vi "Lighthouse Monitoring & Control System with addtional features DONE(GUI LEFT).vi"() -> ()   [LabVIEW 2012]
uses:
  <vilib>/DAQmx/read.llb/DAQmx Read (Counter DBL 1Chan 1Samp).vi
  <vilib>/DAQmx/write.llb/DAQmx Write (Analog DBL 1Chan 1Samp).vi
  <vilib>/DAQmx/write.llb/DAQmx Write (Digital U8 1Chan 1Samp).vi
  <vilib>/DAQmx/write.llb/DAQmx Write (Digital 1D Bool NChan 1Samp 1Line).vi
  <vilib>/DAQmx/read.llb/DAQmx Read (Analog DBL 1Chan 1Samp).vi
  <vilib>/DAQmx/create/channels.llb/DAQmx Create Channel (CI-Count Edges).vi
  <vilib>/DAQmx/create/channels.llb/DAQmx Create Channel (DO-Digital Output).vi
  <vilib>/DAQmx/create/channels.llb/DAQmx Create Channel (AI-Voltage-Basic).vi
  <vilib>/DAQmx/create/channels.llb/DAQmx Create Channel (AO-Voltage-Basic).vi
  <vilib>/DAQmx/miscellaneous.llb/DAQmx Fill In Error Info.vi
panel:
  out "Voltage":dbl
  out "Slot Count":dbl
  out "Data to Write":u32=255 format="%x"
  out "Motor":bool[](array[boolean])
  out "LED 3":bool
  out "LED 2":bool
  out "LED 1":bool
  in  "?":bool
  in  "Switch":bool
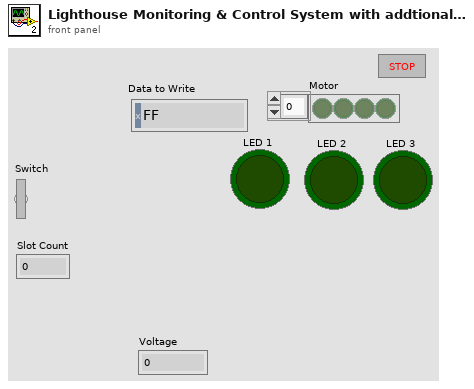
[diagram p1: front panel]
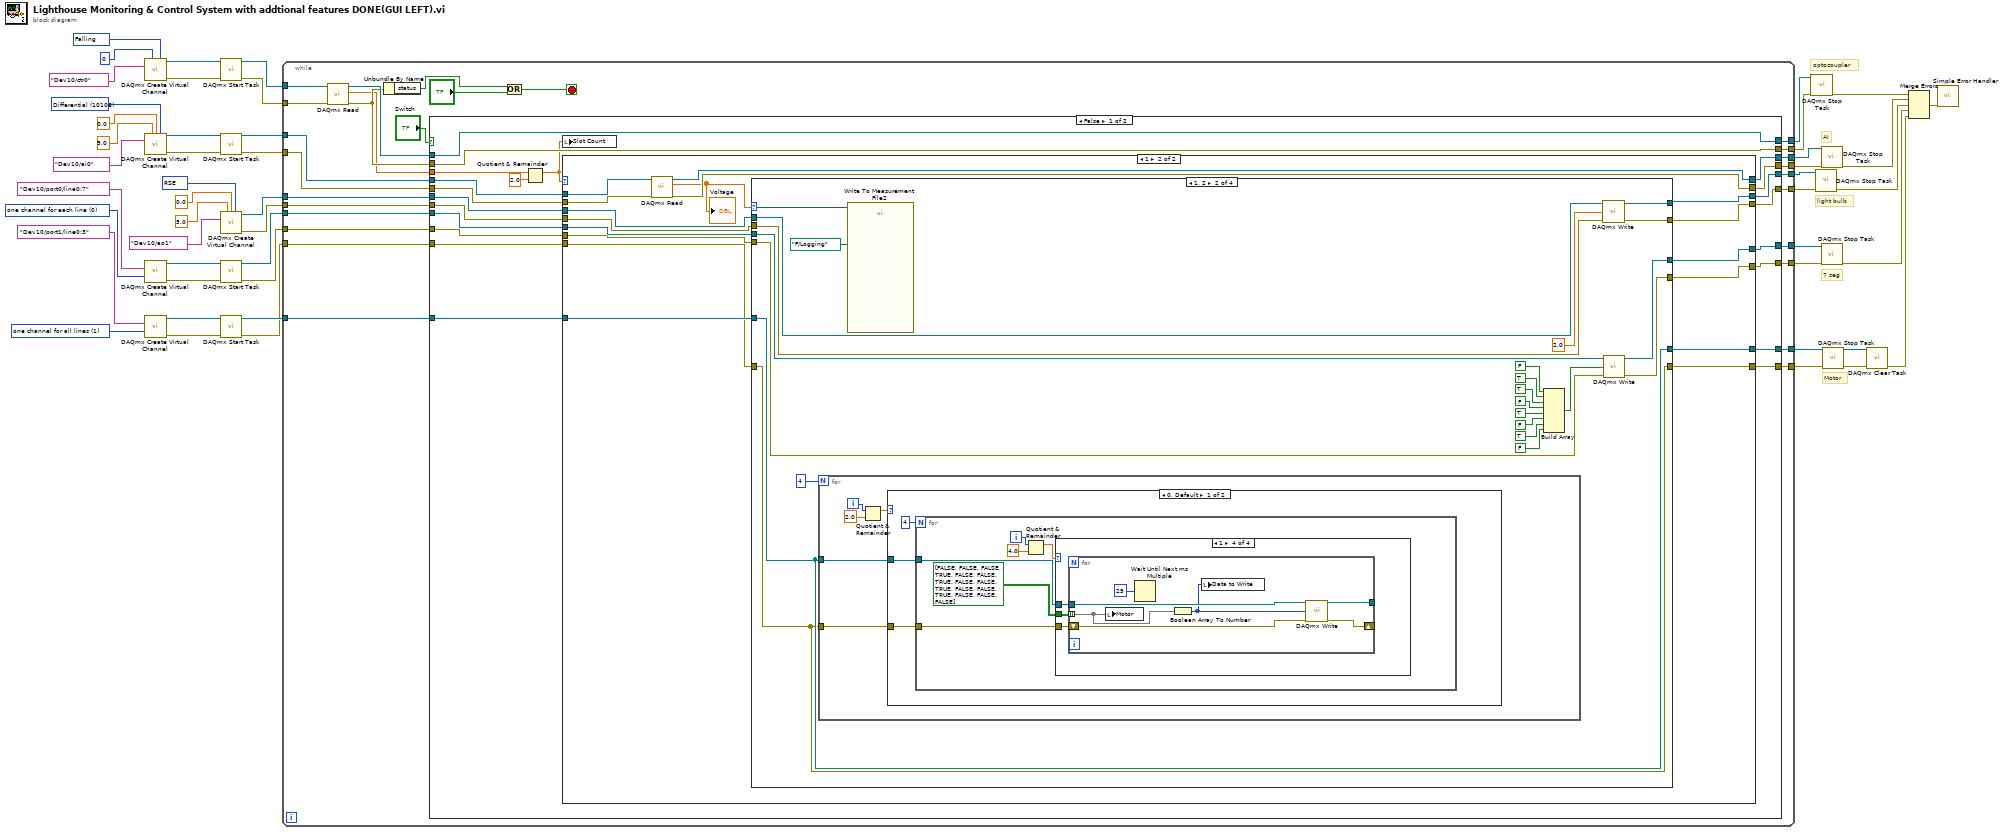
[diagram p0: block diagram]
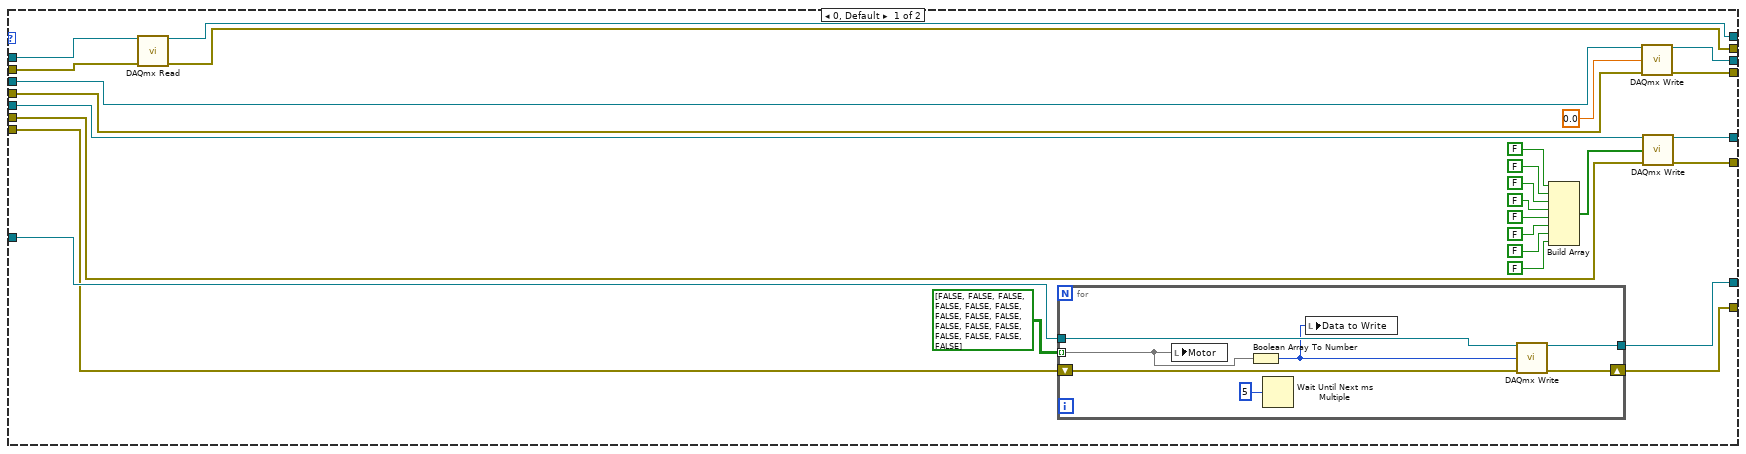
[diagram p2: hidden frame]
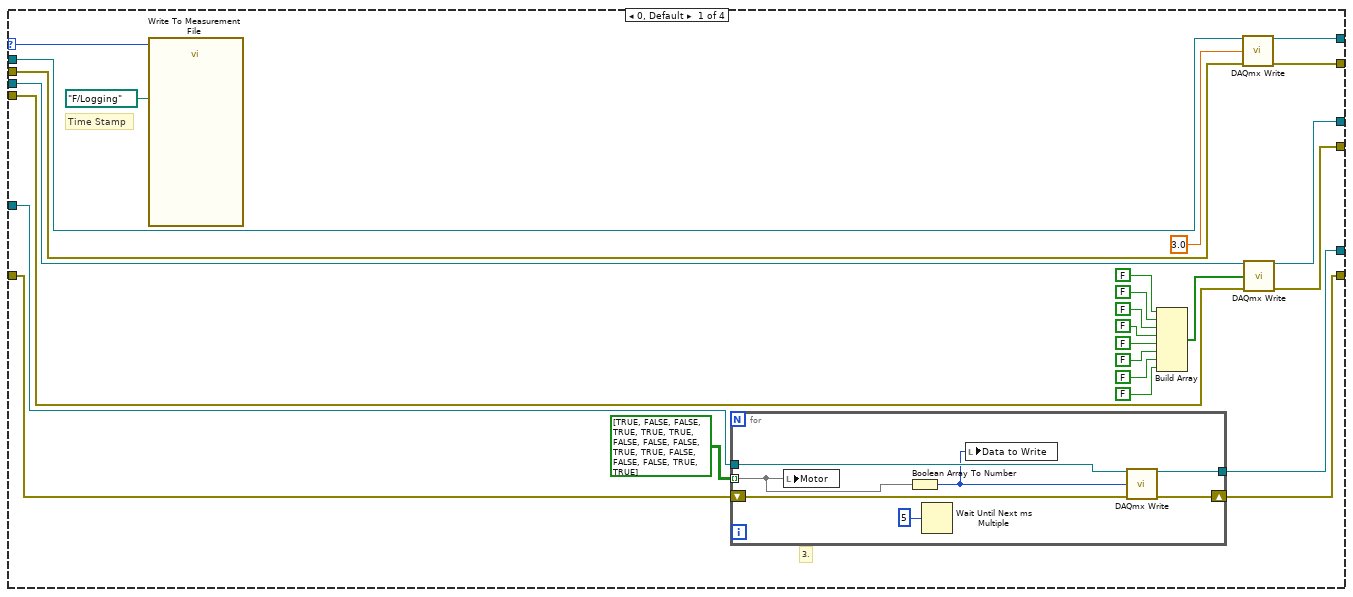
[diagram p3: hidden frame]
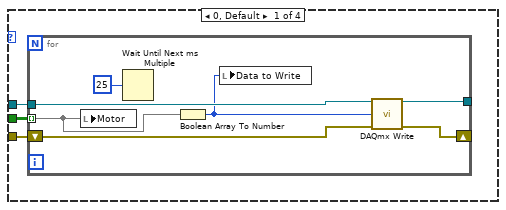
[diagram p4: hidden frame]
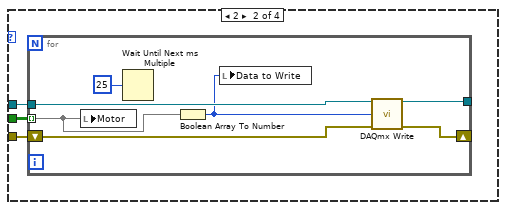
[diagram p5: hidden frame]
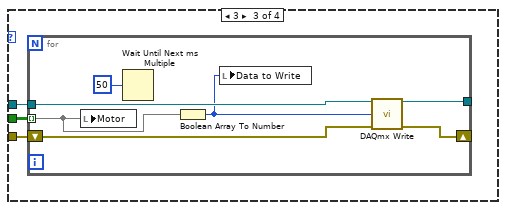
[diagram p6: hidden frame]
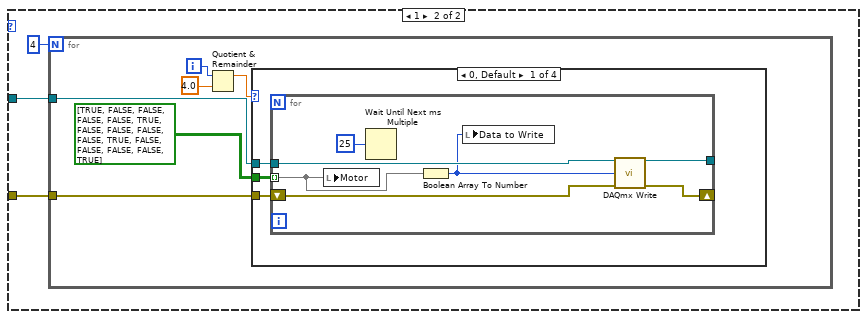
[diagram p7: hidden frame]
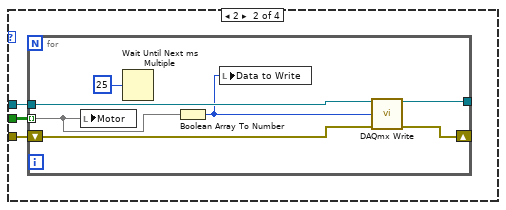
[diagram p8: hidden frame]
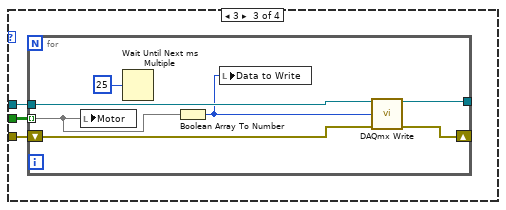
[diagram p9: hidden frame]
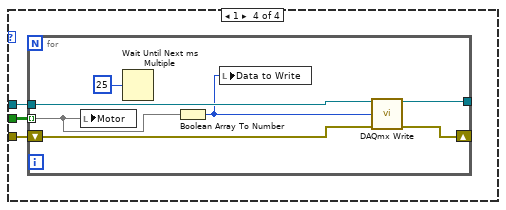
[diagram p10: hidden frame]
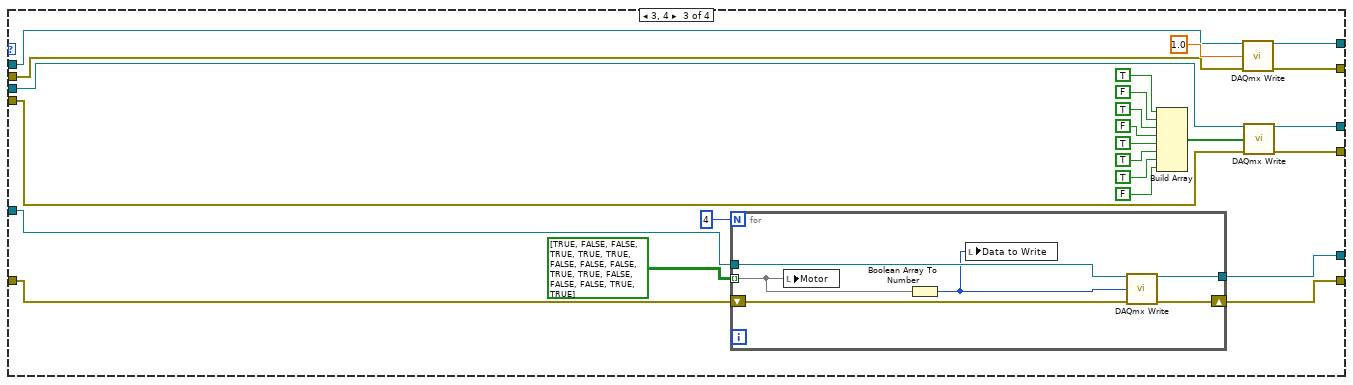
[diagram p11: hidden frame]
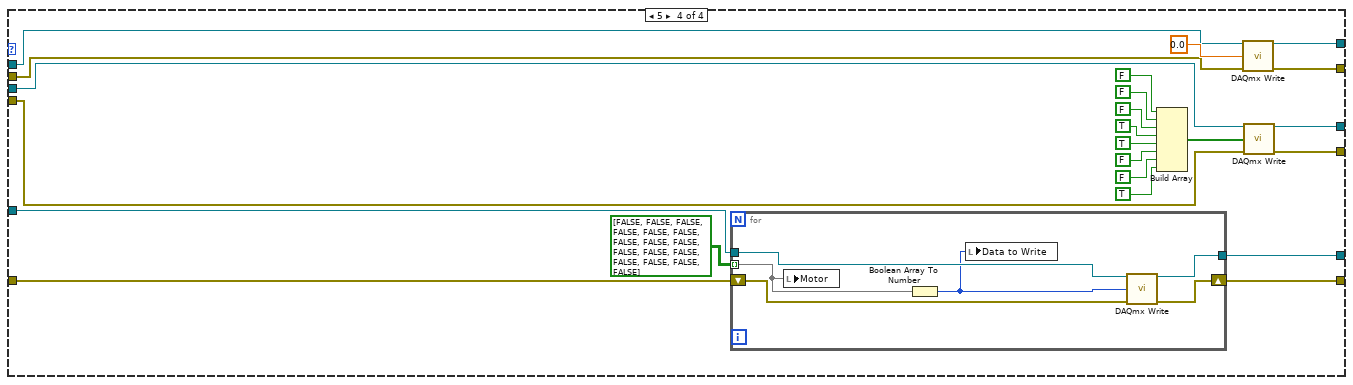
[diagram p12: hidden frame]
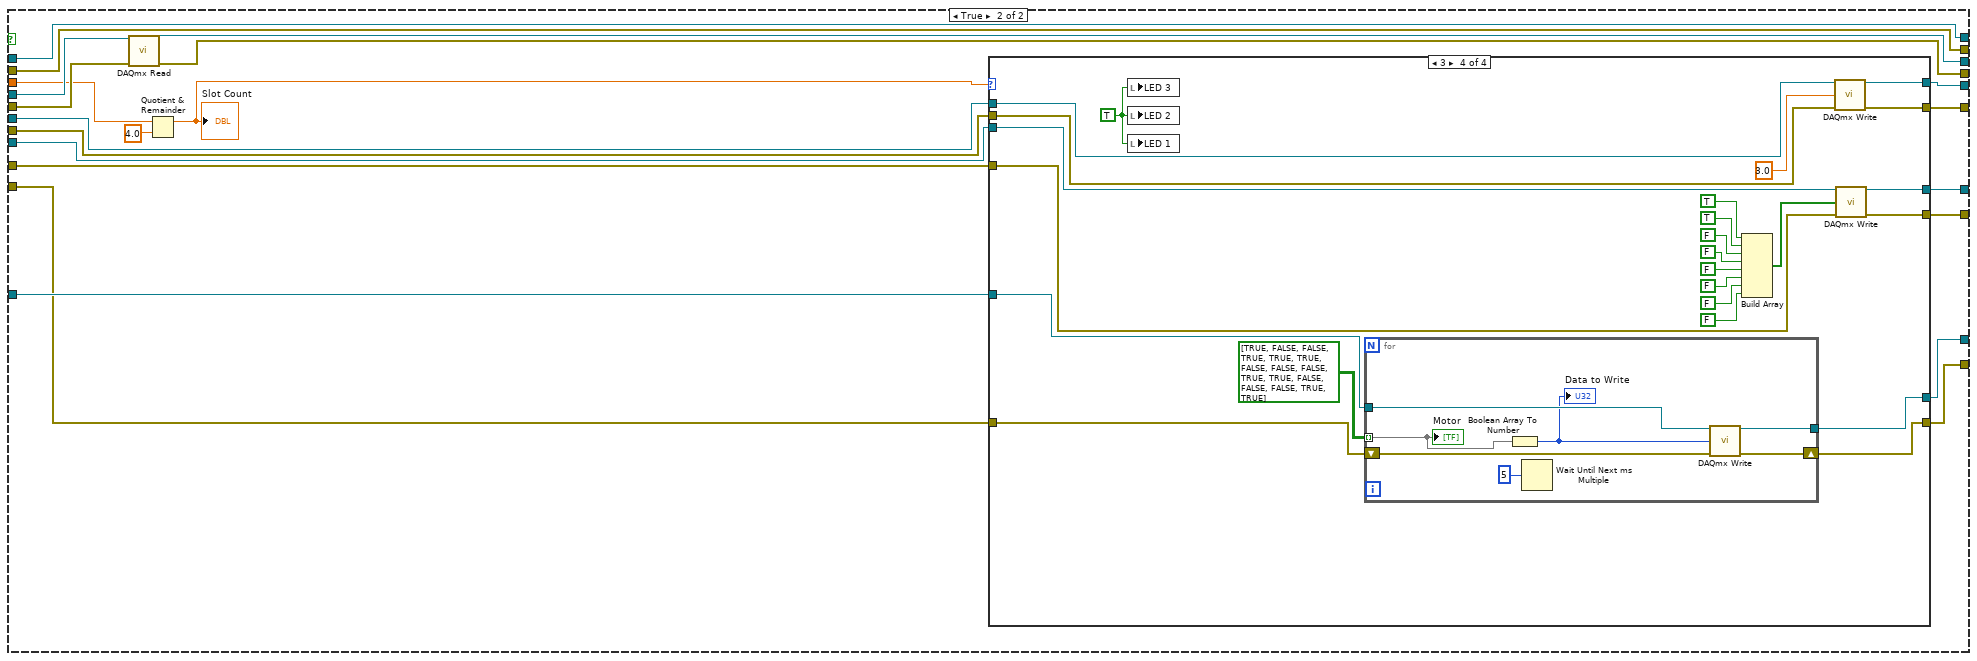
[diagram p13: hidden frame]
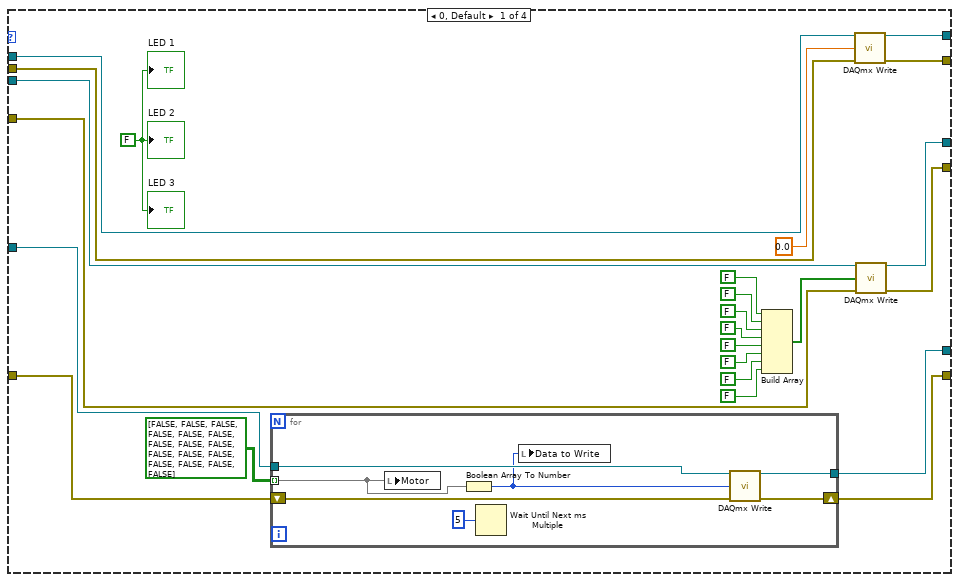
[diagram p14: hidden frame]
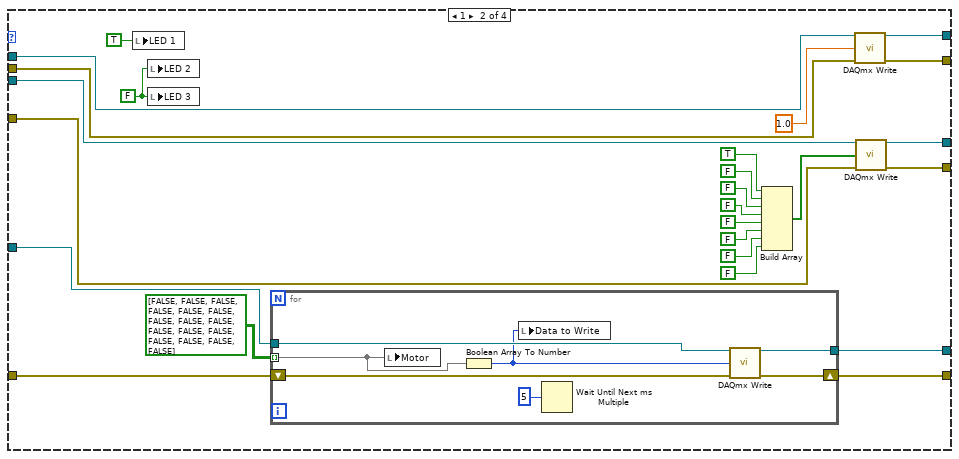
[diagram p15: hidden frame]
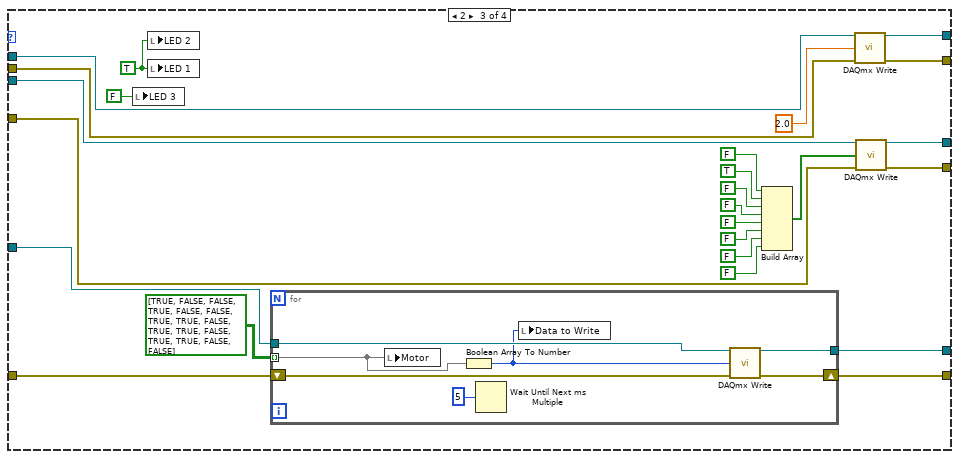
[diagram p16: hidden frame]
diagram:
  w24 = 10083 items=["Default"=-1, "RSE"=10083, "Differential"=10106, "Pseudodifferential"=12529] ("output terminal configuration")
  w32 = 10106 items=["default"=-1, "RSE"=10083, "NRSE"=10078, "Differential"=10106, "Pseudodifferential"=12529] ("input terminal configuration")
  w42 = 1 items=["one channel for each line", "one channel for all lines"] ("line grouping")
  w37 = 0 items=["one channel for each line", "one channel for all lines"] ("line grouping")
  w51 = 10171 items=["Rising"=10280, "Falling"=10171] ("edge")
  # "Motor"
  # "7 seg"
  # "AI"
  # "light bulb"
  # "optocoupler"
  n1 = call-poly <vilib>:"DAQmx Create Virtual Channel.vi"("initial count"=u32 0, "edge"=w51, "counter"=tag "Dev10/ctr0") -> ("task out"=w50:refnum<k21>, "error out"=w49:errorcluster)  [unwired: 11 in]
  n2 = call-poly <vilib>:"DAQmx Create Virtual Channel.vi"("maximum value"=5.0, "minimum value"=0.0, "input terminal configuration"=w32, "physical channels"=tag "Dev10/ai0") -> ("task out"=w30:refnum<k21>, "error out"=w31:errorcluster)  [unwired: 10 in]
  n3 = call-poly <vilib>:"DAQmx Create Virtual Channel.vi"("lines"=tag "Dev10/port0/line0:7", "line grouping"=w37) -> ("task out"=w44:refnum<k21>, "error out"=w43:errorcluster)  [unwired: 12 in]
  n4 = call-poly <vilib>:"DAQmx Create Virtual Channel.vi"("lines"=tag "Dev10/port1/line0:3", "line grouping"=w42) -> ("task out"=w41:refnum<k21>, "error out"=w40:errorcluster)  [unwired: 12 in]
  n5 = call <vilib>:"DAQmx Start Task.vi"("task/channels in"=w50, "error in"=w49) -> ("task out"=w46:refnum<k21>, "error out"=w45:errorcluster)  [unwired: 12 in]
  n6 = call <vilib>:"DAQmx Start Task.vi"("task/channels in"=w30, "error in"=w31) -> ("task out"=w26:refnum<k21>, "error out"=w25:errorcluster)  [unwired: 12 in]
  n7 = call-poly <vilib>:"DAQmx Create Virtual Channel.vi"("maximum value"=5.0, "minimum value"=0.0, "output terminal configuration"=w24, "physical channels"=tag "Dev10/ao1") -> ("task out"=w20:refnum<k21>, "error out"=w19:errorcluster)  [unwired: 10 in]
  n8 = call <vilib>:"DAQmx Start Task.vi"("task/channels in"=w44, "error in"=w43) -> ("task out"=w36:refnum<k21>, "error out"=w35:errorcluster)  [unwired: 12 in]
  n9 = call <vilib>:"DAQmx Start Task.vi"("task/channels in"=w41, "error in"=w40) -> ("task out"=w34:refnum<k21>, "error out"=w33:errorcluster)  [unwired: 12 in]
  n10 = while {
    tunnel: w46 -> [w77]
    tunnel: w45 -> [w76]
    tunnel: w36 -> [w75]
    tunnel: w35 -> [w74]
    tunnel: w34 -> [w73]
    tunnel: w33 -> [w72]
    tunnel: w26 -> [w70]
    tunnel: w25 -> [w69]
    tunnel: w20 -> [w68]
    tunnel: w19 -> [w67]
    tunnel: [w61] -> w10
    tunnel: [w60] -> w9
    tunnel: [w59] -> w8
    tunnel: [w58] -> w7
    tunnel: [w57] -> w6
    tunnel: [w56] -> w5
    tunnel: [w55] -> w4
    tunnel: [w54] -> w3
    tunnel: [w53] -> w2
    tunnel: [w52] -> w1
    stop <- w62 stop-if-true
    n11 = call-poly <vilib>:"DAQmx Read.vi"("task/channels in"=w77, "error in"=w76) -> ("task out"=w65:refnum<k21>, "data"=w63:dbl, "error out"=w64:errorcluster)  [unwired: 11 in]
    n12 = Unbundle By Name(w64) -> ("status"=w71:bool)
    n13 = case shown="False" "Switch" {
      tunnel: w75 -> [w87 w388]
      tunnel: w74 -> [w86 w387]
      tunnel: w73 -> [w85 w386]
      tunnel: w72 -> [w84 w385]
      tunnel: [w83 w384] -> w55
      tunnel: [w82 w383] -> w54
      tunnel: w70 -> [w97 w380]
      tunnel: w69 -> [w96 w379]
      tunnel: w68 -> [w81 w382]
      tunnel: w67 -> [w80 w381]
      tunnel: [w95 w378] -> w53
      tunnel: [w94 w377] -> w52
      tunnel: [w93 w376] -> w59
      tunnel: [w92 w375] -> w58
      tunnel: [w89 w374] -> w56
      tunnel: [w88 w373] -> w57
      tunnel: w65 -> [w91 w369]
      tunnel: w64 -> [w90 w368]
      tunnel: w63 -> [w98 w371]
      tunnel: [w91 w369] -> w61
      tunnel: [w90 w368] -> w60
      frame False {
        n14 = Quotient & Remainder(x=w98, y=2.0) -> (x-y*floor(x/y)=w79:dbl)  [unwired: 1 out]
        n15 = local write "Slot Count"(w79) -> ()
        n16 = case shown="1" w79 {
          tunnel: w97 -> [w125 w150]
          tunnel: w96 -> [w124 w149]
          tunnel: [w121 w148] -> w93
          tunnel: [w122 w147] -> w92
          tunnel: [w123 w146] -> w94
          tunnel: [w118 w145] -> w89
          tunnel: [w119 w144] -> w88
          tunnel: [w120 w143] -> w95
          tunnel: [w106 w141] -> w82
          tunnel: [w107 w142] -> w83
          tunnel: w87 -> [w105 w135]
          tunnel: w86 -> [w104 w134]
          tunnel: w85 -> [w103 w137]
          tunnel: w84 -> [w102 w136]
          tunnel: w81 -> [w101 w139]
          tunnel: w80 -> [w100 w138]
          frame 0, Default {
            n17 = call-poly <vilib>:"DAQmx Read.vi"("task/channels in"=w125, "error in"=w124) -> ("task out"=w120:refnum<k21>, "error out"=w123:errorcluster)  [unwired: 11 in, 1 out]
            n18 = for {
              tunnel: [w132] -> w107
              shift-right: [w130] -> w106
              shift-left: w102 -> [w133]
              tunnel: bool[][] [[FALSE, FALSE, FALSE, FALSE], [FALSE, FALSE, FALSE, FALSE], [FALSE, FALSE, FALSE, FALSE], [FALSE, FALSE, FALSE, FALSE]] -> [w127] mode=indexing
              tunnel: w103 -> [w129]
              n19 = local write "Motor"(w127) -> ()
              n20 = Boolean Array To Number(Boolean array=w127) -> (number=w128:u32)
              n21 = Wait Until Next ms Multiple(millisecond multiple=5) -> ()  [unwired: 1 out]
              n22 = local write "Data to Write"(w128) -> ()
              n23 = call-poly <vilib>:"DAQmx Write.vi"("task/channels in"=w129, "data"=w128, "error in"=w133) -> ("task out"=w132:refnum<k21>, "error out"=w130:errorcluster)  [unwired: 10 in, 1 out]
            }
            n24 = Build Array(FALSE, FALSE, FALSE, FALSE, FALSE, FALSE, FALSE, FALSE) -> (w109:bool[])
            n25 = call-poly <vilib>:"DAQmx Write.vi"("task/channels in"=w101, "data"=0.0, "error in"=w100) -> ("task out"=w121:refnum<k21>, "error out"=w122:errorcluster)  [unwired: 10 in, 1 out]
            n26 = call-poly <vilib>:"DAQmx Write.vi"("task/channels in"=w105, "data"=w109, "error in"=w104) -> ("task out"=w119:refnum<k21>, "error out"=w118:errorcluster)  [unwired: 10 in, 1 out]
          }
          frame 1 {
            n27 = call-poly <vilib>:"DAQmx Read.vi"("task/channels in"=w150, "error in"=w149) -> ("task out"=w143:refnum<k21>, "data"=w140:dbl, "error out"=w146:errorcluster)  [unwired: 11 in]
            "Voltage" <- w140
            n28 = case shown="1, 2" w140 {
              selector: w140 -> [w157 w190 _ _]
              tunnel: [w165 w195 w322 w351] -> w148
              tunnel: [w164 w194 w321 w350] -> w147
              tunnel: [w163 w193 w320 w349] -> w144
              tunnel: [w162 w192 w319 w348] -> w145
              tunnel: [w161 w184 w317 w346] -> w142
              tunnel: [w160 w183 w316 w345] -> w141
              tunnel: w139 -> [w156 w189 w315 w344]
              tunnel: w138 -> [w155 w188 w314 w343]
              tunnel: w137 -> [w154 w184 w311 w340]
              tunnel: w136 -> [w151 w183 w310 w339]
              tunnel: w135 -> [w153 w187 w313 w342]
              tunnel: w134 -> [w152 w186 w312 w341]
              frame 0, Default {
                # "3."
                # "Time Stamp"
                n29 = call "Write To Measurement File"("Signals"=w157, "Filename"=path "F:/Logging") -> ()  [unwired: 15 in, 3 out]
                n30 = for {
                  tunnel: [w181] -> w161
                  shift-right: [w180] -> w160
                  shift-left: w151 -> [w182]
                  tunnel: bool[][] [[TRUE, FALSE, FALSE, TRUE], [TRUE, TRUE, FALSE, FALSE], [FALSE, TRUE, TRUE, FALSE], [FALSE, FALSE, TRUE, TRUE]] -> [w176] mode=indexing
                  tunnel: w154 -> [w178]
                  n31 = local write "Motor"(w176) -> ()
                  n32 = Boolean Array To Number(Boolean array=w176) -> (number=w177:u32)
                  n33 = Wait Until Next ms Multiple(millisecond multiple=u32 5) -> ()  [unwired: 1 out]
                  n34 = local write "Data to Write"(w177) -> ()
                  n35 = call-poly <vilib>:"DAQmx Write.vi"("task/channels in"=w178, "data"=w177, "error in"=w182) -> ("task out"=w181:refnum<k21>, "error out"=w180:errorcluster)  [unwired: 10 in, 1 out]
                }
                n36 = Build Array(FALSE, FALSE, FALSE, FALSE, FALSE, FALSE, FALSE, FALSE) -> (w166:bool[])
                n37 = call-poly <vilib>:"DAQmx Write.vi"("task/channels in"=w156, "data"=3.0, "error in"=w155) -> ("task out"=w165:refnum<k21>, "error out"=w164:errorcluster)  [unwired: 10 in, 1 out]
                n38 = call-poly <vilib>:"DAQmx Write.vi"("task/channels in"=w153, "data"=w166, "error in"=w152) -> ("task out"=w163:refnum<k21>, "error out"=w162:errorcluster)  [unwired: 10 in, 1 out]
              }
              frame 1, 2 {
                n39 = for {
                  N: 4 -> [_]
                  tunnel: w184 -> [w210]
                  tunnel: w183 -> [w209]
                  i -> [w207]
                  n40 = Quotient & Remainder(x=w207, y=2.0) -> (x-y*floor(x/y)=w206:dbl)  [unwired: 1 out]
                  n41 = case shown="0, Default" w206 {
                    tunnel: w210 -> [w213 w262]
                    tunnel: w209 -> [w212 w261]
                    frame 0, Default {
                      n42 = for {
                        N: 4 -> [_]
                        tunnel: w213 -> [w219]
                        tunnel: w212 -> [w218]
                        i -> [w215]
                        n43 = Quotient & Remainder(x=w215, y=4.0) -> (x-y*floor(x/y)=w214:dbl)  [unwired: 1 out]
                        n44 = case shown="1" w214 {
                          tunnel: w219 -> [w222 w232 w241 w252]
                          tunnel: w218 -> [w220 w231 w242 w251]
                          tunnel: bool[][] [[FALSE, FALSE, FALSE, TRUE], [FALSE, FALSE, TRUE, FALSE], [FALSE, TRUE, FALSE, FALSE], [TRUE, FALSE, FALSE, FALSE]] -> [w221 w230 w240 w250]
                          frame 0, Default {
                            n45 = for {
                              tunnel: [w228] -> _
                              shift-right: [w227] -> _
                              shift-left: w220 -> [w229]
                              tunnel: w221 -> [w223] mode=indexing
                              tunnel: w222 -> [w225]
                              n46 = local write "Motor"(w223) -> ()
                              n47 = Wait Until Next ms Multiple(millisecond multiple=u32 25) -> ()  [unwired: 1 out]
                              n48 = Boolean Array To Number(Boolean array=w223) -> (number=w224:u32)
                              n49 = local write "Data to Write"(w224) -> ()
                              n50 = call-poly <vilib>:"DAQmx Write.vi"("task/channels in"=w225, "data"=w224, "error in"=w229) -> ("task out"=w228:refnum<k21>, "error out"=w227:errorcluster)  [unwired: 10 in, 1 out]
                            }
                          }
                          frame 2 {
                            n51 = for {
                              tunnel: [w238] -> _
                              shift-right: [w237] -> _
                              shift-left: w231 -> [w239]
                              tunnel: w230 -> [w233] mode=indexing
                              tunnel: w232 -> [w235]
                              n52 = local write "Motor"(w233) -> ()
                              n53 = Wait Until Next ms Multiple(millisecond multiple=u32 25) -> ()  [unwired: 1 out]
                              n54 = Boolean Array To Number(Boolean array=w233) -> (number=w234:u32)
                              n55 = local write "Data to Write"(w234) -> ()
                              n56 = call-poly <vilib>:"DAQmx Write.vi"("task/channels in"=w235, "data"=w234, "error in"=w239) -> ("task out"=w238:refnum<k21>, "error out"=w237:errorcluster)  [unwired: 10 in, 1 out]
                            }
                          }
                          frame 3 {
                            n57 = for {
                              tunnel: [w248] -> _
                              shift-right: [w247] -> _
                              shift-left: w242 -> [w249]
                              tunnel: w240 -> [w244] mode=indexing
                              tunnel: w241 -> [w245]
                              n58 = local write "Motor"(w244) -> ()
                              n59 = Wait Until Next ms Multiple(millisecond multiple=u32 50) -> ()  [unwired: 1 out]
                              n60 = Boolean Array To Number(Boolean array=w244) -> (number=w243:u32)
                              n61 = local write "Data to Write"(w243) -> ()
                              n62 = call-poly <vilib>:"DAQmx Write.vi"("task/channels in"=w245, "data"=w243, "error in"=w249) -> ("task out"=w248:refnum<k21>, "error out"=w247:errorcluster)  [unwired: 10 in, 1 out]
                            }
                          }
                          frame 1 {
                            n63 = for {
                              tunnel: [w258] -> _
                              shift-right: [w257] -> _
                              shift-left: w251 -> [w259]
                              tunnel: w250 -> [w254] mode=indexing
                              tunnel: w252 -> [w255]
                              n64 = local write "Motor"(w254) -> ()
                              n65 = Wait Until Next ms Multiple(millisecond multiple=u32 25) -> ()  [unwired: 1 out]
                              n66 = Boolean Array To Number(Boolean array=w254) -> (number=w253:u32)
                              n67 = local write "Data to Write"(w253) -> ()
                              n68 = call-poly <vilib>:"DAQmx Write.vi"("task/channels in"=w255, "data"=w253, "error in"=w259) -> ("task out"=w258:refnum<k21>, "error out"=w257:errorcluster)  [unwired: 10 in, 1 out]
                            }
                          }
                        }
                      }
                    }
                    frame 1 {
                      n69 = for {
                        N: 4 -> [_]
                        tunnel: w262 -> [w268]
                        tunnel: w261 -> [w267]
                        i -> [w266]
                        n70 = Quotient & Remainder(x=w266, y=4.0) -> (x-y*floor(x/y)=w264:dbl)  [unwired: 1 out]
                        n71 = case shown="0, Default" w264 {
                          tunnel: w268 -> [w271 w281 w290 w301]
                          tunnel: w267 -> [w270 w280 w291 w300]
                          tunnel: bool[][] [[TRUE, FALSE, FALSE, FALSE], [FALSE, TRUE, FALSE, FALSE], [FALSE, FALSE, TRUE, FALSE], [FALSE, FALSE, FALSE, TRUE]] -> [w269 w279 w289 w299]
                          frame 0, Default {
                            n72 = for {
                              tunnel: [w277] -> _
                              shift-right: [w276] -> _
                              shift-left: w270 -> [w278]
                              tunnel: w269 -> [w273] mode=indexing
                              tunnel: w271 -> [w274]
                              n73 = local write "Motor"(w273) -> ()
                              n74 = Wait Until Next ms Multiple(millisecond multiple=u32 25) -> ()  [unwired: 1 out]
                              n75 = Boolean Array To Number(Boolean array=w273) -> (number=w272:u32)
                              n76 = local write "Data to Write"(w272) -> ()
                              n77 = call-poly <vilib>:"DAQmx Write.vi"("task/channels in"=w274, "data"=w272, "error in"=w278) -> ("task out"=w277:refnum<k21>, "error out"=w276:errorcluster)  [unwired: 10 in, 1 out]
                            }
                          }
                          frame 2 {
                            n78 = for {
                              tunnel: [w287] -> _
                              shift-right: [w286] -> _
                              shift-left: w280 -> [w288]
                              tunnel: w279 -> [w282] mode=indexing
                              tunnel: w281 -> [w284]
                              n79 = local write "Motor"(w282) -> ()
                              n80 = Wait Until Next ms Multiple(millisecond multiple=u32 25) -> ()  [unwired: 1 out]
                              n81 = Boolean Array To Number(Boolean array=w282) -> (number=w283:u32)
                              n82 = local write "Data to Write"(w283) -> ()
                              n83 = call-poly <vilib>:"DAQmx Write.vi"("task/channels in"=w284, "data"=w283, "error in"=w288) -> ("task out"=w287:refnum<k21>, "error out"=w286:errorcluster)  [unwired: 10 in, 1 out]
                            }
                          }
                          frame 3 {
                            n84 = for {
                              tunnel: [w297] -> _
                              shift-right: [w296] -> _
                              shift-left: w291 -> [w298]
                              tunnel: w289 -> [w293] mode=indexing
                              tunnel: w290 -> [w294]
                              n85 = local write "Motor"(w293) -> ()
                              n86 = Wait Until Next ms Multiple(millisecond multiple=u32 25) -> ()  [unwired: 1 out]
                              n87 = Boolean Array To Number(Boolean array=w293) -> (number=w292:u32)
                              n88 = local write "Data to Write"(w292) -> ()
                              n89 = call-poly <vilib>:"DAQmx Write.vi"("task/channels in"=w294, "data"=w292, "error in"=w298) -> ("task out"=w297:refnum<k21>, "error out"=w296:errorcluster)  [unwired: 10 in, 1 out]
                            }
                          }
                          frame 1 {
                            n90 = for {
                              tunnel: [w307] -> _
                              shift-right: [w306] -> _
                              shift-left: w300 -> [w308]
                              tunnel: w299 -> [w303] mode=indexing
                              tunnel: w301 -> [w304]
                              n91 = local write "Motor"(w303) -> ()
                              n92 = Wait Until Next ms Multiple(millisecond multiple=u32 25) -> ()  [unwired: 1 out]
                              n93 = Boolean Array To Number(Boolean array=w303) -> (number=w302:u32)
                              n94 = local write "Data to Write"(w302) -> ()
                              n95 = call-poly <vilib>:"DAQmx Write.vi"("task/channels in"=w304, "data"=w302, "error in"=w308) -> ("task out"=w307:refnum<k21>, "error out"=w306:errorcluster)  [unwired: 10 in, 1 out]
                            }
                          }
                        }
                      }
                    }
                  }
                }
                n96 = call "Write To Measurement File2"("Signals"=w190, "Filename"=path "F:/Logging") -> ()  [unwired: 15 in, 3 out]
                n97 = Build Array(FALSE, TRUE, TRUE, FALSE, TRUE, FALSE, TRUE, FALSE) -> (w196:bool[])
                n98 = call-poly <vilib>:"DAQmx Write.vi"("task/channels in"=w189, "data"=2.0, "error in"=w188) -> ("task out"=w195:refnum<k21>, "error out"=w194:errorcluster)  [unwired: 10 in, 1 out]
                n99 = call-poly <vilib>:"DAQmx Write.vi"("task/channels in"=w187, "data"=w196, "error in"=w186) -> ("task out"=w193:refnum<k21>, "error out"=w192:errorcluster)  [unwired: 10 in, 1 out]
              }
              frame 3, 4 {
                n100 = for {
                  N: 4 -> [_]
                  tunnel: [w337] -> w317
                  shift-right: [w336] -> w316
                  shift-left: w310 -> [w338]
                  tunnel: bool[][] [[TRUE, FALSE, FALSE, TRUE], [TRUE, TRUE, FALSE, FALSE], [FALSE, TRUE, TRUE, FALSE], [FALSE, FALSE, TRUE, TRUE]] -> [w333] mode=indexing
                  tunnel: w311 -> [w335]
                  n101 = local write "Motor"(w333) -> ()
                  n102 = Boolean Array To Number(Boolean array=w333) -> (number=w334:u32)
                  n103 = local write "Data to Write"(w334) -> ()
                  n104 = call-poly <vilib>:"DAQmx Write.vi"("task/channels in"=w335, "data"=w334, "error in"=w338) -> ("task out"=w337:refnum<k21>, "error out"=w336:errorcluster)  [unwired: 10 in, 1 out]
                }
                n105 = Build Array(TRUE, FALSE, TRUE, FALSE, TRUE, TRUE, TRUE, FALSE) -> (w323:bool[])
                n106 = call-poly <vilib>:"DAQmx Write.vi"("task/channels in"=w315, "data"=1.0, "error in"=w314) -> ("task out"=w322:refnum<k21>, "error out"=w321:errorcluster)  [unwired: 10 in, 1 out]
                n107 = call-poly <vilib>:"DAQmx Write.vi"("task/channels in"=w313, "data"=w323, "error in"=w312) -> ("task out"=w320:refnum<k21>, "error out"=w319:errorcluster)  [unwired: 10 in, 1 out]
              }
              frame 5 {
                n108 = for {
                  tunnel: [w366] -> w346
                  shift-right: [w365] -> w345
                  shift-left: w339 -> [w367]
                  tunnel: bool[][] [[FALSE, FALSE, FALSE, FALSE], [FALSE, FALSE, FALSE, FALSE], [FALSE, FALSE, FALSE, FALSE], [FALSE, FALSE, FALSE, FALSE]] -> [w362] mode=indexing
                  tunnel: w340 -> [w364]
                  n109 = local write "Motor"(w362) -> ()
                  n110 = Boolean Array To Number(Boolean array=w362) -> (number=w363:u32)
                  n111 = local write "Data to Write"(w363) -> ()
                  n112 = call-poly <vilib>:"DAQmx Write.vi"("task/channels in"=w364, "data"=w363, "error in"=w367) -> ("task out"=w366:refnum<k21>, "error out"=w365:errorcluster)  [unwired: 10 in, 1 out]
                }
                n113 = Build Array(FALSE, FALSE, FALSE, TRUE, TRUE, FALSE, FALSE, TRUE) -> (w352:bool[])
                n114 = call-poly <vilib>:"DAQmx Write.vi"("task/channels in"=w344, "data"=0.0, "error in"=w343) -> ("task out"=w351:refnum<k21>, "error out"=w350:errorcluster)  [unwired: 10 in, 1 out]
                n115 = call-poly <vilib>:"DAQmx Write.vi"("task/channels in"=w342, "data"=w352, "error in"=w341) -> ("task out"=w349:refnum<k21>, "error out"=w348:errorcluster)  [unwired: 10 in, 1 out]
              }
            }
          }
        }
      }
      frame True {
        n116 = call-poly <vilib>:"DAQmx Read.vi"("task/channels in"=w380, "error in"=w379) -> ("task out"=w378:refnum<k21>, "error out"=w377:errorcluster)  [unwired: 11 in, 1 out]
        n117 = Quotient & Remainder(x=w371, y=4.0) -> (x-y*floor(x/y)=w370:dbl)  [unwired: 1 out]
        "Slot Count" <- w370
        n118 = case shown="3" w370 {
          tunnel: w388 -> [w400 w428 w460 w491]
          tunnel: w387 -> [w399 w427 w461 w492]
          tunnel: w386 -> [w412 w426 w457 w489]
          tunnel: w385 -> [w411 w425 w458 w488]
          tunnel: [w410 w424 w456 w487] -> w384
          tunnel: [w409 w423 w455 w486] -> w383
          tunnel: w382 -> [w397 w439 w473 w504]
          tunnel: w381 -> [w396 w438 w472 w503]
          tunnel: [w395 w441 w475 w506] -> w376
          tunnel: [w394 w440 w474 w505] -> w375
          tunnel: [w391 w421 w453 w485] -> w373
          tunnel: [w390 w420 w452 w484] -> w374
          frame 0, Default {
            w392 = FALSE
            n119 = for {
              tunnel: [w418] -> w410
              shift-right: [w416] -> w409
              shift-left: w411 -> [w419]
              tunnel: w412 -> [w415]
              tunnel: bool[][] [[FALSE, FALSE, FALSE, FALSE], [FALSE, FALSE, FALSE, FALSE], [FALSE, FALSE, FALSE, FALSE], [FALSE, FALSE, FALSE, FALSE]] -> [w413] mode=indexing
              n120 = local write "Motor"(w413) -> ()
              n121 = Boolean Array To Number(Boolean array=w413) -> (number=w414:u32)
              n122 = Wait Until Next ms Multiple(millisecond multiple=5) -> ()  [unwired: 1 out]
              n123 = local write "Data to Write"(w414) -> ()
              n124 = call-poly <vilib>:"DAQmx Write.vi"("task/channels in"=w415, "data"=w414, "error in"=w419) -> ("task out"=w418:refnum<k21>, "error out"=w416:errorcluster)  [unwired: 10 in, 1 out]
            }
            n125 = Build Array(FALSE, FALSE, FALSE, FALSE, FALSE, FALSE, FALSE, FALSE) -> (w401:bool[])
            n126 = call-poly <vilib>:"DAQmx Write.vi"("task/channels in"=w397, "data"=0.0, "error in"=w396) -> ("task out"=w395:refnum<k21>, "error out"=w394:errorcluster)  [unwired: 10 in, 1 out]
            n127 = call-poly <vilib>:"DAQmx Write.vi"("task/channels in"=w400, "data"=w401, "error in"=w399) -> ("task out"=w391:refnum<k21>, "error out"=w390:errorcluster)  [unwired: 10 in, 1 out]
            "LED 1" <- w392
            "LED 2" <- w392
            "LED 3" <- w392
          }
          frame 1 {
            w444 = FALSE ("LED 2")
            n128 = local write "LED 1"(TRUE ("LED 1")) -> ()
            n129 = local write "LED 2"(w444) -> ()
            n130 = local write "LED 3"(w444) -> ()
            n131 = for {
              tunnel: [w450] -> w424
              shift-right: [w448] -> w423
              shift-left: w425 -> [w451]
              tunnel: w426 -> [w447]
              tunnel: bool[][] [[FALSE, FALSE, FALSE, FALSE], [FALSE, FALSE, FALSE, FALSE], [FALSE, FALSE, FALSE, FALSE], [FALSE, FALSE, FALSE, FALSE]] -> [w446] mode=indexing
              n132 = local write "Motor"(w446) -> ()
              n133 = Boolean Array To Number(Boolean array=w446) -> (number=w445:u32)
              n134 = local write "Data to Write"(w445) -> ()
              n135 = Wait Until Next ms Multiple(millisecond multiple=5) -> ()  [unwired: 1 out]
              n136 = call-poly <vilib>:"DAQmx Write.vi"("task/channels in"=w447, "data"=w445, "error in"=w451) -> ("task out"=w450:refnum<k21>, "error out"=w448:errorcluster)  [unwired: 10 in, 1 out]
            }
            n137 = Build Array(TRUE, FALSE, FALSE, FALSE, FALSE, FALSE, FALSE, FALSE) -> (w429:bool[])
            n138 = call-poly <vilib>:"DAQmx Write.vi"("task/channels in"=w439, "data"=1.0, "error in"=w438) -> ("task out"=w441:refnum<k21>, "error out"=w440:errorcluster)  [unwired: 10 in, 1 out]
            n139 = call-poly <vilib>:"DAQmx Write.vi"("task/channels in"=w428, "data"=w429, "error in"=w427) -> ("task out"=w421:refnum<k21>, "error out"=w420:errorcluster)  [unwired: 10 in, 1 out]
          }
          frame 2 {
            w471 = TRUE ("LED 2")
            n140 = local write "LED 3"(FALSE ("LED 3")) -> ()
            n141 = local write "LED 2"(w471) -> ()
            n142 = local write "LED 1"(w471) -> ()
            n143 = for {
              tunnel: [w482] -> w456
              shift-right: [w480] -> w455
              shift-left: w458 -> [w483]
              tunnel: w457 -> [w479]
              tunnel: bool[][] [[TRUE, FALSE, FALSE, TRUE], [FALSE, FALSE, TRUE, TRUE], [FALSE, TRUE, TRUE, FALSE], [TRUE, TRUE, FALSE, FALSE]] -> [w477] mode=indexing
              n144 = local write "Motor"(w477) -> ()
              n145 = Boolean Array To Number(Boolean array=w477) -> (number=w478:u32)
              n146 = Wait Until Next ms Multiple(millisecond multiple=5) -> ()  [unwired: 1 out]
              n147 = local write "Data to Write"(w478) -> ()
              n148 = call-poly <vilib>:"DAQmx Write.vi"("task/channels in"=w479, "data"=w478, "error in"=w483) -> ("task out"=w482:refnum<k21>, "error out"=w480:errorcluster)  [unwired: 10 in, 1 out]
            }
            n149 = Build Array(FALSE ("element"), TRUE, FALSE, FALSE, FALSE, FALSE, FALSE, FALSE) -> (w462:bool[])
            n150 = call-poly <vilib>:"DAQmx Write.vi"("task/channels in"=w473, "data"=2.0, "error in"=w472) -> ("task out"=w475:refnum<k21>, "error out"=w474:errorcluster)  [unwired: 10 in, 1 out]
            n151 = call-poly <vilib>:"DAQmx Write.vi"("task/channels in"=w460, "data"=w462, "error in"=w461) -> ("task out"=w453:refnum<k21>, "error out"=w452:errorcluster)  [unwired: 10 in, 1 out]
          }
          frame 3 {
            w502 = TRUE ("LED 3")
            n152 = local write "LED 3"(w502) -> ()
            n153 = local write "LED 2"(w502) -> ()
            n154 = local write "LED 1"(w502) -> ()
            n155 = for {
              tunnel: [w513] -> w487
              shift-right: [w511] -> w486
              shift-left: w488 -> [w514]
              tunnel: w489 -> [w510]
              tunnel: bool[][] [[TRUE, FALSE, FALSE, TRUE], [TRUE, TRUE, FALSE, FALSE], [FALSE, TRUE, TRUE, FALSE], [FALSE, FALSE, TRUE, TRUE]] -> [w508] mode=indexing
              n156 = Boolean Array To Number(Boolean array=w508) -> (number=w509:u32)
              "Data to Write" <- w509
              n157 = Wait Until Next ms Multiple(millisecond multiple=5) -> ()  [unwired: 1 out]
              n158 = call-poly <vilib>:"DAQmx Write.vi"("task/channels in"=w510, "data"=w509, "error in"=w514) -> ("task out"=w513:refnum<k21>, "error out"=w511:errorcluster)  [unwired: 10 in, 1 out]
              "Motor" <- w508
            }
            n159 = Build Array(TRUE, TRUE, FALSE, FALSE, FALSE, FALSE, FALSE, FALSE) -> (w493:bool[])
            n160 = call-poly <vilib>:"DAQmx Write.vi"("task/channels in"=w504, "data"=3.0, "error in"=w503) -> ("task out"=w506:refnum<k21>, "error out"=w505:errorcluster)  [unwired: 10 in, 1 out]
            n161 = call-poly <vilib>:"DAQmx Write.vi"("task/channels in"=w491, "data"=w493, "error in"=w492) -> ("task out"=w485:refnum<k21>, "error out"=w484:errorcluster)  [unwired: 10 in, 1 out]
          }
        }
      }
    }
    n162 = Or(x=w71, y="?") -> (x .or. y?=w62:bool)
  }
  n163 = call <vilib>:"DAQmx Stop Task.vi"("task/channels in"=w10, "error in"=w9) -> ("error out"=w18:errorcluster)  [unwired: 12 in, 1 out]
  n164 = call <vilib>:"DAQmx Stop Task.vi"("task/channels in"=w8, "error in"=w7) -> ("error out"=w16:errorcluster)  [unwired: 12 in, 1 out]
  n165 = call <vilib>:"DAQmx Stop Task.vi"("task/channels in"=w2, "error in"=w1) -> ("error out"=w17:errorcluster)  [unwired: 12 in, 1 out]
  n166 = call <vilib>:"DAQmx Stop Task.vi"("task/channels in"=w6, "error in"=w5) -> ("error out"=w15:errorcluster)  [unwired: 12 in, 1 out]
  n167 = call <vilib>:"DAQmx Stop Task.vi"("task/channels in"=w4, "error in"=w3) -> ("task out"=w13:refnum<k21>, "error out"=w12:errorcluster)  [unwired: 12 in]
  n168 = call <vilib>:"DAQmx Clear Task.vi"("task in"=w13, "error in"=w12) -> ("error out"=w11:errorcluster)  [unwired: 13 in]
  n169 = Merge Errors(w18, w17, w16, w15, w11) -> (w14:errorcluster)
  n170 = call <vilib>:"Simple Error Handler.vi"("error in (no error)"=w14) -> ()  [unwired: 4 in, 5 out]
